vi "简易流程路径读取.vi"(8 "error in (no error)":errorcluster caption="错误输入（无错误）", 11 "Cleaningcycle 输入":refnum<class "Cleaning cycle.lvclass">) -> (0 "error out":errorcluster caption="错误输出", 2 "简易流程路径":path, 3 "Cleaningcycle 输出":refnum<class "Cleaning cycle.lvclass">)   [LabVIEW 2022 SP3, in "Cleaning cycle.lvclass"]
uses:
  Cleaning cycle.lvclass
  Cleaning cycle.lvclass/Cleaning cycle.ctl
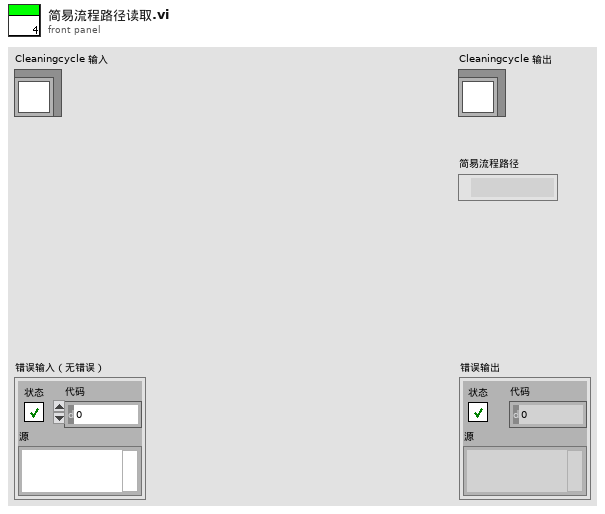
[diagram p1: front panel]
types:
  T1 = typedef "Cleaning cycle.lvclass/State Data.ctl" = cluster{"配置文件路径":path, "简易流程路径":path, "参数列表":cluster{"String":string, "Value":u16}[], "简易流程列表":cluster{"String":string, "Value":u16}[], "配置信息":T2, "命令":cluster{"触发":bool, "周期项":T4}[]}
  T2 = typedef "Cleaning cycle.lvclass/配置信息.ctl" = cluster{"任务列表":T3}
  T3 = typedef "Cleaning cycle.lvclass/任务.ctl" = cluster{"启用":bool, "项":string[][]}
  T4 = typedef "Cleaning cycle.lvclass/周期项.ctl" = cluster{"时":i32, "分":i32, "频次":string, "id":i32, "参数":string, "simpleflowid":i32, "简易流程名称":string}
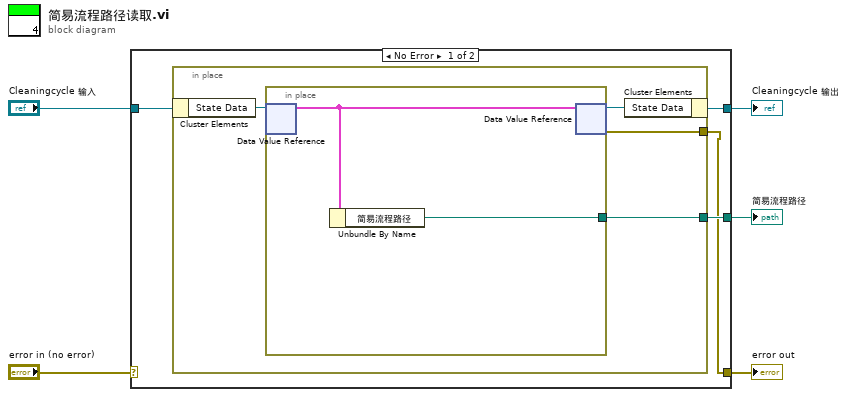
[diagram p0: block diagram]
diagram:
  n1 = case shown="No Error" "error in (no error)" {
    selector: "error in (no error)" -> [_ w17]
    tunnel: [w6 w17] -> w4
    tunnel: [w8 w16] -> w2
    tunnel: "Cleaningcycle 输入" -> [w9 w16]
    tunnel: [w7 _] -> w1
    frame No Error {
      n2 = in-place {
        in-place-border: [w11] -> w7
        in-place-border: [w10] -> w6
        n3 = in-place-cluster #1(w9) -> ("State Data"=w13:refnum<data-value>)
        n4 = in-place {
          in-place-border: [w14] -> w11
          n5 = in-place-dvr #2(w13) -> (w15:T1)  [unwired: 1 out]
          n6 = Unbundle By Name(w15) -> ("简易流程路径"=w14:path)
          n7 = in-place-dvr #2(w15) -> (w12:refnum<data-value>, w10:errorcluster)
        }
        n8 = in-place-cluster #1("State Data"=w12) -> (w8:refnum<class "Cleaning cycle.lvclass">)
      }
    }
    frame Error {
    }
  }
  "error out" <- w4
  "Cleaningcycle 输出" <- w2
  "简易流程路径" <- w1
